vi "Pie Fourths.vi"(1 "Input":dbl) -> (0 "Output":dbl)   [LabVIEW 2015]
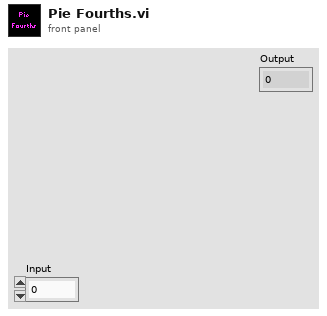
[diagram p1: front panel]
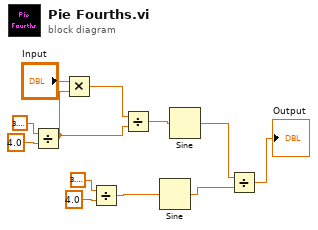
[diagram p0: block diagram]
diagram:
  n1 = Divide(x=3.141592653589793, y=4.0) -> (x/y=w5:dbl)
  n2 = Multiply(x="Input", y=w5) -> (x*y=w4:dbl)
  n3 = Divide(x=3.141592653589793, y=4.0) -> (x/y=w6:dbl)
  n4 = Divide(x=w4, y=w5) -> (x/y=w9:dbl)
  n5 = Sine(x=w6) -> (sin(x)=w3:dbl)
  n6 = Sine(x=w9) -> (sin(x)=w2:dbl)
  n7 = Divide(x=w2, y=w3) -> (x/y=→"Output":dbl)
